vi "InitialConditionTest.vi"(11 "error in":errorcluster) -> (15 "error out":errorcluster)   [LabVIEW 2016]
uses:
  Car Wash 16.0/Controls/Wash Options.ctl
  Car Wash 16.0/Controls/Car Wash Indicators.ctl
  Car Wash 16.0/Car Wash.vi
  main/apis/Setup/GetVI/GetVIByPath.vi
  main/apis/Assert/AssertControlValueCompare/AssertControlValueEqual.vi
  main/apis/Stimulus/ValueSignalByPathString.vi
  <vilib>/addons/_JKI Toolkits/Caraya/classes/Test/Test.lvclass
  Car Wash 16.0/Car Wash.lvlib
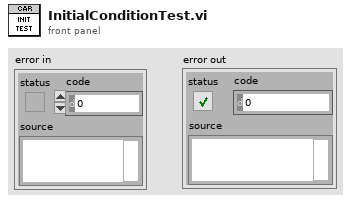
[diagram p1: front panel]
types:
  T1 = enum32{"Invalid", "Standard", "Closed", "Hidden", "Minimized", "Maximized"}
  T2 = typedef "Car Wash.lvlib/Car Wash Indicators.ctl" = cluster{"Underbody Wash":bool, "Bug Remover":bool, "Pre-Soak":bool, "High Pressure Wash":bool, "Low Pressure Wax":bool, "Spot Free Rinse":bool, "Tire Shine Foam":bool, "Air Dry":bool, "Vehicle Out of Position":bool}
  T3 = typedef "Car Wash.lvlib/Wash Options.ctl" = cluster{"Underbody Wash":bool, "Bug Remover":bool, "Pre-Soak":bool, "High Pressure Wash":bool, "Low Pressure Wax":bool, "Spot Free Rinse":bool, "Tire Shine Foam":bool, "Air Dry":bool}
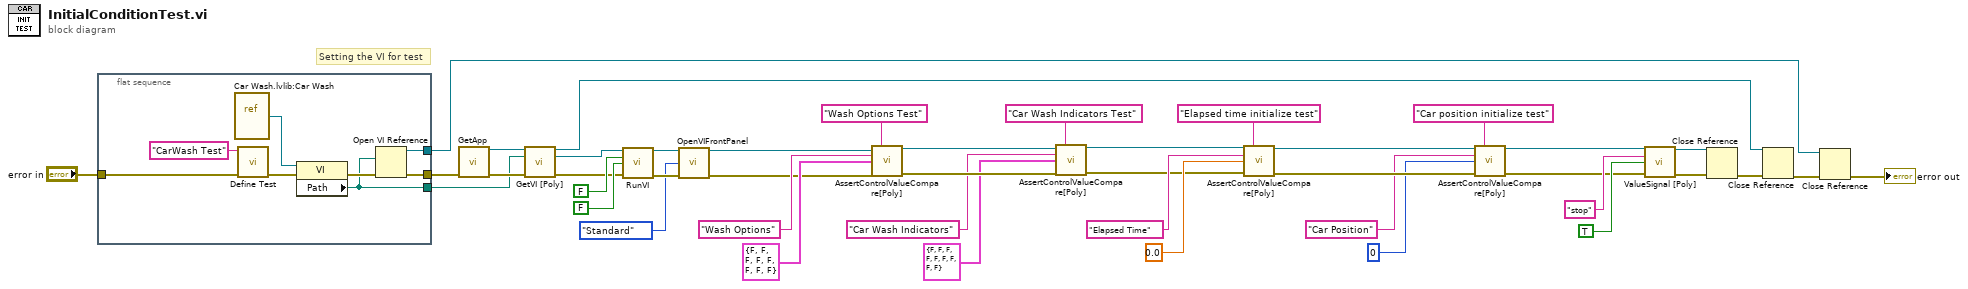
[diagram p0: block diagram]
diagram:
  # "Setting the VI for test"
  n1 = flat-sequence {
    tunnel: [w48] -> w25
    tunnel: [w47] -> w3
    tunnel: [w45] -> w20
    tunnel: "error in" -> [w44]
    frame #0 {
      n2 = vi-ref "Car Wash.lvlib:Car Wash.vi"() -> (w50:refnum<vi>)
      n3 = call <vilib>:"Define Test.vi"("error in (no error)"=w44, "Label (VI Title)"="CarWash Test") -> ("error out"=w51:errorcluster)  [unwired: 9 in]
      n4 = property on="Property Node" class="VI"(reference=w50, error in=w51) -> (error out=w49:errorcluster, "Path"=w45:path)  [unwired: 1 out]
      n5 = Open VI Reference(vi path=w45, error in (no error)=w49) -> (vi reference=w47:refnum<vi>, error out=w48:errorcluster)  [unwired: 4 in]
    }
  }
  n6 = call "GetApp.vi"("error in (no error)"=w25) -> ("Application Ref"=w21:refnum<vi>, "error out"=w22:errorcluster)  [unwired: 13 in]
  n7 = call-poly "GetVI [Poly].vi"("Application Ref in"=w21, "VI Path"=w20, "error in (no error)"=w22) -> ("Application Ref out"=w4:refnum<vi>, "VI Reference"=w19:refnum<vi>, "error out"=w18:errorcluster)  [unwired: 10 in]
  n8 = call "RunVI.vi"("VI Reference In"=w19, "Wait Until Done (F)"=FALSE ("Wait Until Done"), "Auto Dispose Reference (F)"=FALSE ("Auto Dispose Reference"), "error in"=w18) -> ("VI Reference Out"=w16:refnum<vi>, "error out"=w17:errorcluster)  [unwired: 10 in]
  n9 = call "OpenVIFrontPanel.vi"("VI Reference In"=w16, "State"=T1."Standard", "error in"=w17) -> ("VI Reference Out"=w5:refnum<vi>, "error out"=w15:errorcluster)  [unwired: 11 in]
  n10 = call-poly "AssertControlValueCompare[Poly].vi"("VI Reference In"=w5, "Label"="Wash Options Test", "Control Name"="Wash Options", "Control Value"=T3 {"Underbody Wash"=FALSE, "Bug Remover"=FALSE, "Pre-Soak"=FALSE, "High Pressure Wash"=FALSE, "Low Pressure Wax"=FALSE, "Spot Free Rinse"=FALSE, "Tire Shine Foam"=FALSE, "Air Dry"=FALSE} ("Wash Options"), "error out"=w15) -> ("VI Reference Out"=w29:refnum<vi>, "error out"=w32:errorcluster)  [unwired: 9 in]
  n11 = call-poly "AssertControlValueCompare[Poly].vi"("VI Reference In"=w29, "Label"="Car Wash Indicators Test", "Control Name"="Car Wash Indicators", "Control Value"=T2 {"Underbody Wash"=FALSE, "Bug Remover"=FALSE, "Pre-Soak"=FALSE, "High Pressure Wash"=FALSE, "Low Pressure Wax"=FALSE, "Spot Free Rinse"=FALSE, "Tire Shine Foam"=FALSE, "Air Dry"=FALSE, "Vehicle Out of Position"=FALSE} ("Car Wash Indicators"), "error out"=w32) -> ("VI Reference Out"=w30:refnum<vi>, "error out"=w31:errorcluster)  [unwired: 9 in]
  n12 = call-poly "AssertControlValueCompare[Poly].vi"("VI Reference In"=w30, "Label"="Elapsed time initialize test", "Control Name"="Elapsed Time", "Control Value"=0.0, "error out"=w31) -> ("VI Reference Out"=w38:refnum<vi>, "error out"=w39:errorcluster)  [unwired: 9 in]
  n13 = call-poly "AssertControlValueCompare[Poly].vi"("VI Reference In"=w38, "Label"="Car position initialize test", "Control Name"="Car Position", "Control Value"=u8 0, "error out"=w39) -> ("VI Reference Out"=w6:refnum<vi>, "error out"=w7:errorcluster)  [unwired: 9 in]
  n14 = call-poly "ValueSignal [Poly].vi"("VI Reference In"=w6, "Control Name"="stop", "Value (Signaling)"=TRUE, "error in"=w7) -> ("VI Reference Out"=w10:refnum<vi>, "error out"=w12:errorcluster)  [unwired: 10 in]
  n15 = Close Reference(reference=w10, error in (no error)=w12) -> (error out=w11:errorcluster)
  n16 = Close Reference(reference=w4, error in (no error)=w11) -> (error out=w9:errorcluster)
  n17 = Close Reference(reference=w3, error in (no error)=w9) -> (error out=→"error out":errorcluster)
